vi "SerialEngine.vi"() -> ()   [LabVIEW 2011]
uses:
  Tushars Events/Software/Modules/EventClient_ObjectReference.ctl
  Strict Type Controls/Settings Operation.ctl
  <vilib>/Instr/_visa.llb/VISA Configure Serial Port (Instr).vi
panel:
  out "Quit":bool
  out "error out":errorcluster
  in  "error in (no error)":errorcluster
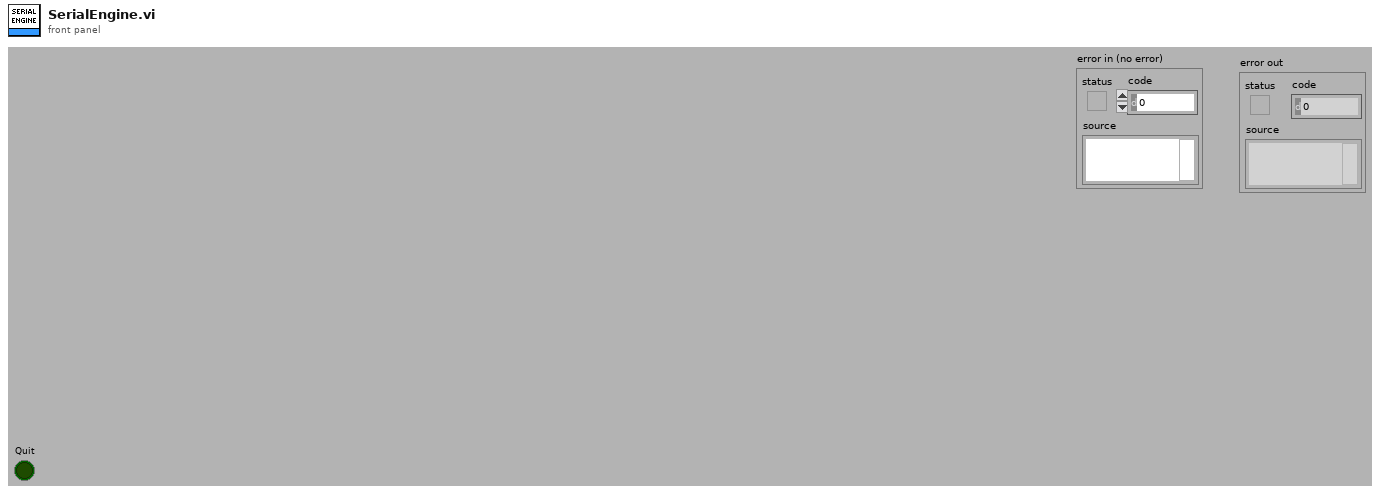
[diagram p1: front panel]
types:
  T1 = typedef "EventClient_ObjectReference.ctl" = refnum<k1>
  T2 = typedef "Settings Operation.ctl" = enum8{"Get Value", "Set Value", "Read File", "Write File", "Write Stored Value"}
  T3 = typedef "Settings.ctl" = cluster{"DMM Settings":cluster{"Port":refnum<visa-resource-name>, "baud rate":u32, "data bits":u16, "stop bits":u16, "parity":enum16{"None", "Odd", "Even", "Mark", "Space"}, "flow control":enum16{"None", "XON/XOFF", "RTS/CTS", "XON/XOFF & RTS/CTS", "DTR/DSR", "XON/XOFF & DTR/DSR"}}, "Modbus Settings":cluster{"Port":refnum<visa-resource-name>, "baud rate":u32, "parity":enum16{"None", "Odd", "Even", "Mark", "Space"}, "flow control":enum16{"None", "XON/XOFF", "RTS/CTS", "XON/XOFF & RTS/CTS", "DTR/DSR", "XON/XOFF & DTR/DSR"}}}
  T4 = enum16{"None", "XON/XOFF", "RTS/CTS", "XON/XOFF & RTS/CTS", "DTR/DSR", "XON/XOFF & DTR/DSR"}
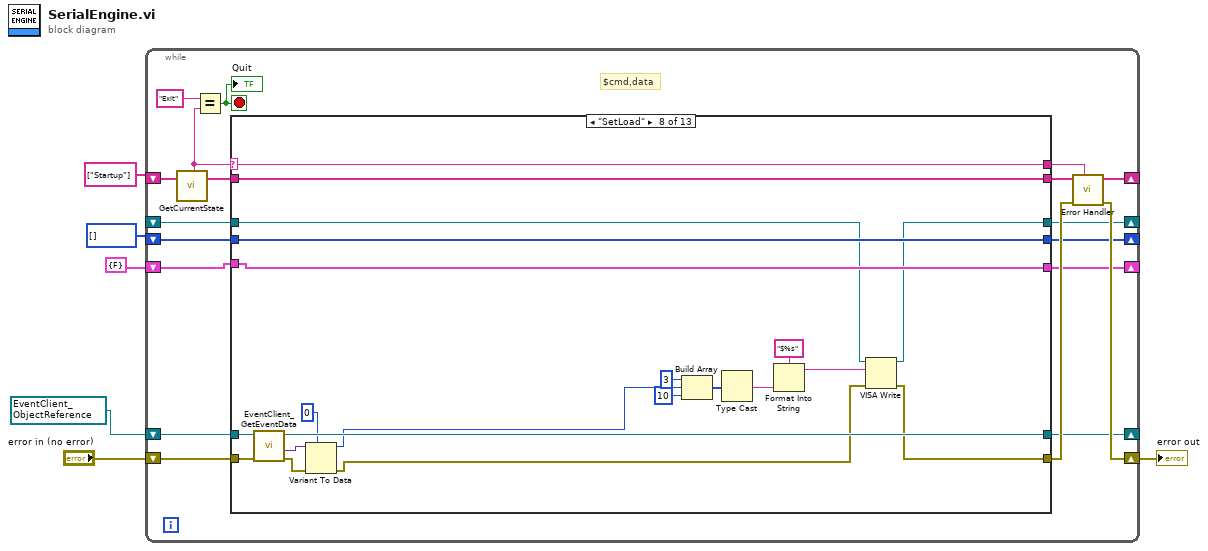
[diagram p0: block diagram]
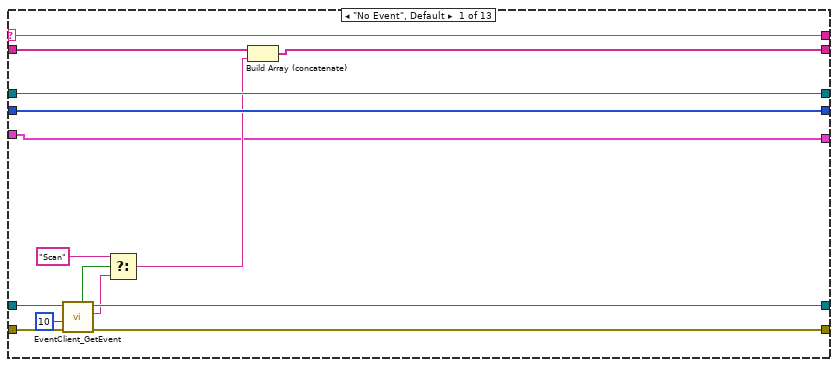
[diagram p2: hidden frame]
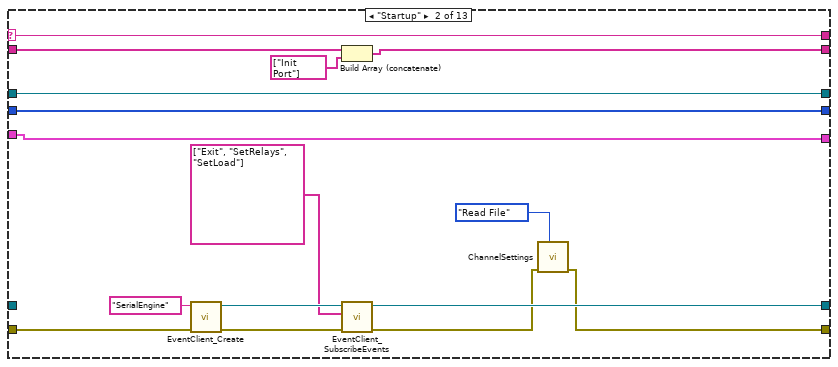
[diagram p3: hidden frame]
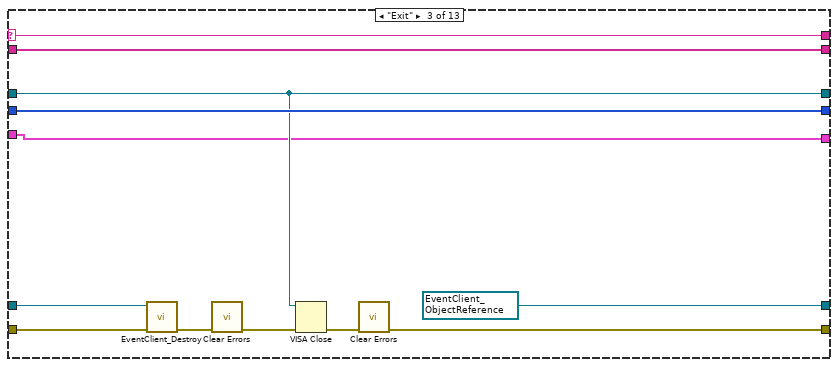
[diagram p4: hidden frame]
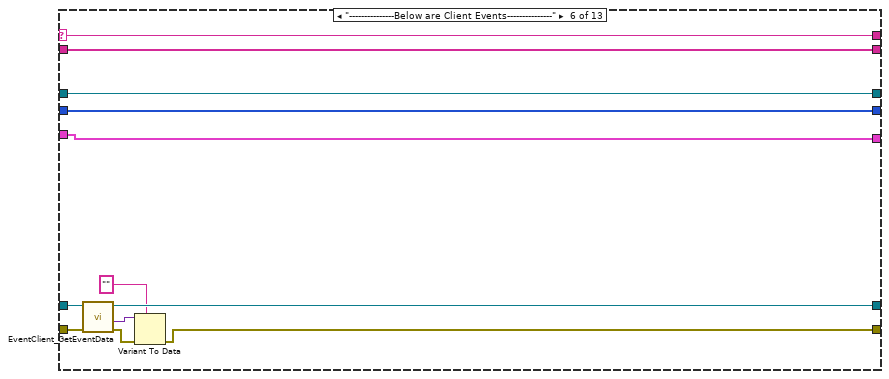
[diagram p7: hidden frame]
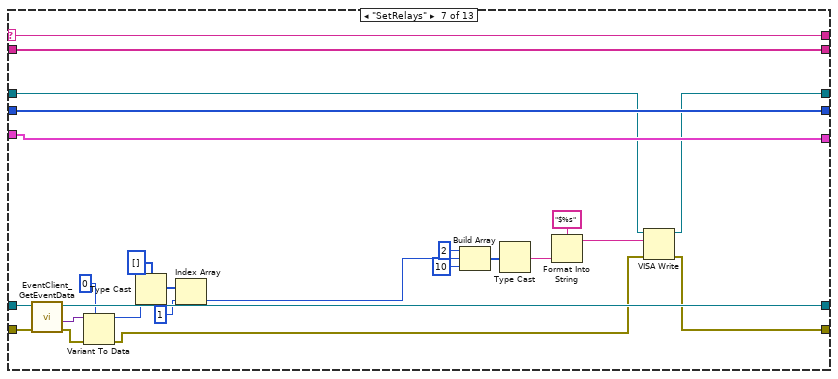
[diagram p8: hidden frame]
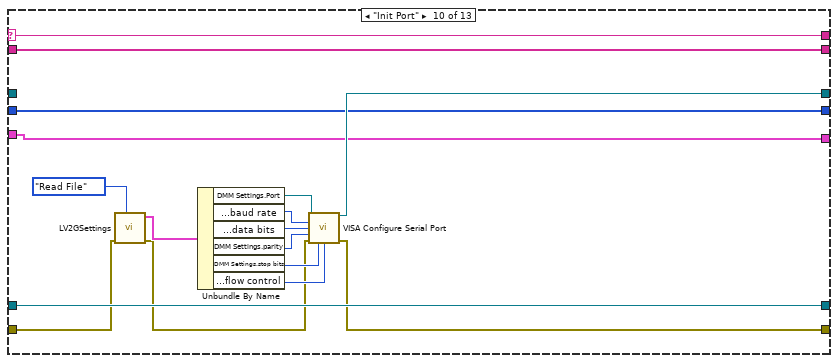
[diagram p10: hidden frame]
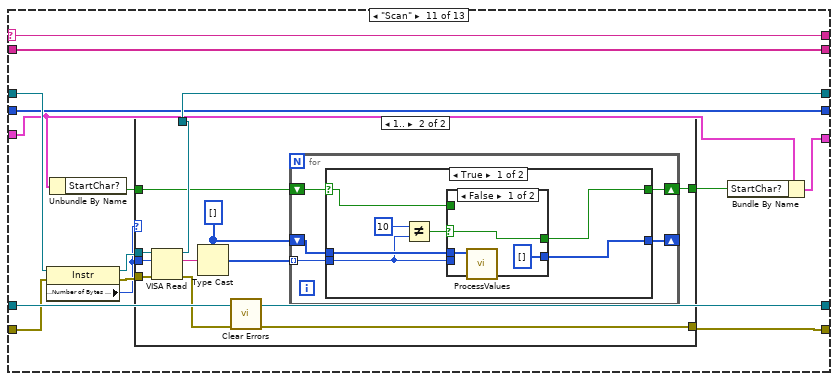
[diagram p11: hidden frame]
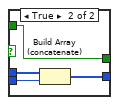
[diagram p13: hidden frame]
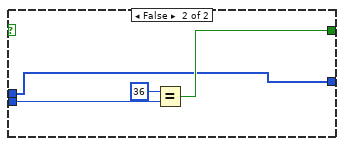
[diagram p14: hidden frame]
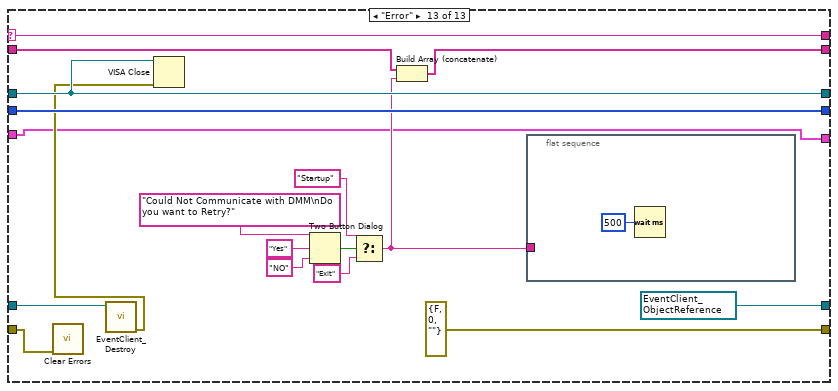
[diagram p16: hidden frame]
diagram:
  w3 = T1 refnum items=["EventClient"] ("reference")
  n1 = while {
    shift-right: [w21] -> _
    shift-left: string[] ["Startup"] ("State Array Out") -> [w25]
    shift-right: [w17] -> w4
    shift-left: "error in (no error)" -> [w18]
    shift-right: [w14] -> _
    shift-left: w3 -> [w13]
    shift-right: [w12] -> _
    shift-left: _ -> [w11]
    shift-right: [w9] -> _
    shift-left: u8[] [] -> [w10]
    shift-right: [w7] -> _
    shift-left: cluster{"StartChar?":bool} {"StartChar?"=FALSE} -> [w8]
    stop <- w22 stop-if-true
    # "$cmd,data"
    n2 = call "GetCurrentState.vi"("State Array In"=w25) -> ("Current State"=w15:string, "State Array Out"=w24:string[])  [unwired: 1 in, 16 out]
    n3 = Equal?(x="Exit", y=w15) -> (x = y?=w22:bool)
    "Quit" <- w22
    n4 = case shown="\"SetLoad\"" w15 {
      selector: w15 -> [w40 w56 w68 w74 w81 w93 w118 w139 w146 w163 w178 w223 w241]
      tunnel: w24 -> [w33 w55 w67 w75 w82 w94 w119 w140 w147 w164 w179 w222 w237]
      tunnel: [w35 w54 w67 w75 w82 w94 w119 w140 w147 w164 w179 w222 w236] -> w20
      tunnel: [w37 w43 w58 w73 w80 w89 w108 w129 w145 w152 w171 w221 errorcluster {"status"=FALSE, "code"=0, "source"=""} ("error in (no error)")] -> w16
      tunnel: [w40 w56 w68 w74 w81 w93 w118 w139 w146 w163 w178 w223 w241] -> w19
      tunnel: w18 -> [w38 w52 w65 w73 w80 w91 w116 w137 w145 w161 w172 w221 w226]
      tunnel: [w36 w49 w64 w72 w79 w87 w113 w134 w144 w162 w177 w220 w227] -> w14
      tunnel: w13 -> [w39 _ w66 w72 w79 w92 w117 w138 w144 w162 w177 w220 w228]
      tunnel: [w32 w46 w62 w71 w78 w86 w106 w127 w143 w151 w173 w219 w238] -> w12
      tunnel: w11 -> [w32 w46 w62 w71 w78 w86 w107 w128 w143 _ w174 w219 w238]
      tunnel: w10 -> [w31 w45 w63 w70 w77 w85 w112 w133 w142 w150 w170 w218 w239]
      tunnel: [w31 w45 w63 w70 w77 w85 w112 w133 w142 w150 w170 w218 w239] -> w9
      tunnel: w8 -> [w26 w41 w57 w69 w76 w83 w111 w132 w141 w149 w167 w217 w224]
      tunnel: [w26 w41 w57 w69 w76 w83 w111 w132 w141 w149 w166 w217 w224] -> w7
      frame "No Event", Default {
        n5 = call "EventClient_GetEvent.vi"("error in (no error)"=w38, "timeout in ms (-1)"=10, "reference"=w39) -> ("error out"=w37:errorcluster, "Name"=w28:string, "reference out"=w36:T1, "timed out?"=w30:bool)  [unwired: 5 out]
        n6 = Select(t="Scan" ("x"), s=w30, f=w28) -> (s? t:f=w27:string)
        n7 = Build Array (concatenate)(w33, w27) -> (w35:string[])
      }
      frame "Startup" {
        n8 = call "EventClient_Create.vi"("error in (no error)"=w52, "Instance Name"="SerialEngine") -> ("error out"=w51:errorcluster, "reference"=w50:T1)  [unwired: 8 out]
        n9 = Build Array (concatenate)(w55, string[] ["Init Port"] ("State Array Out")) -> (w54:string[])
        n10 = call "EventClient_SubscribeEvents.vi"("error in (no error)"=w51, "Events"=string[] ["Exit", "SetRelays", "SetLoad"], "reference"=w50) -> ("error out"=w44:errorcluster, "reference out"=w49:T1)  [unwired: 7 out]
        n11 = call "ChannelSettings.vi"("Operation"=Settings_Operation."Read File", "error in (no error)"=w44) -> ("error out"=w43:errorcluster)  [unwired: 4 in, 4 out]
      }
      frame "Exit" {
        w64 = T1 refnum items=["EventClient"] ("reference out")
        n12 = call "EventClient_Destroy.vi"("error in (no error)"=w65, "reference"=w66) -> ("error out"=w61:errorcluster)  [unwired: 9 out]
        n13 = call <vilib>:"Clear Errors.vi"("error in (no error)"=w61) -> ("error out"=w60:errorcluster)  [unwired: 6 out]
        n14 = VISA Close(VISA resource name=w62, error in (no error)=w60) -> (error out=w59:errorcluster)
        n15 = call <vilib>:"Clear Errors.vi"("error in (no error)"=w59) -> ("error out"=w58:errorcluster)  [unwired: 6 out]
      }
      frame "---------------Below are UI Events---------------" {
        # "This State will never Execute\nIt is added just for improving code readability please do not remove this case"
      }
      frame "---------------Below are Menu Events---------------" {
        # "This State will never Execute\nIt is added just for improving code readability please do not remove this case"
      }
      frame "---------------Below are Client Events---------------" {
        n16 = call "EventClient_GetEventData.vi"("error in (no error)"=w91, "reference"=w92) -> ("error out"=w90:errorcluster, "Data"=w88:variant, "reference out"=w87:T1)  [unwired: 7 out]
        n17 = Variant To Data(error in=w90, type="", Variant=w88) -> (error out=w89:errorcluster)  [unwired: 1 out]
      }
      frame "SetRelays" {
        n18 = call "EventClient_GetEventData.vi"("error in (no error)"=w116, "reference"=w117) -> ("error out"=w115:errorcluster, "Data"=w114:variant, "reference out"=w113:T1)  [unwired: 7 out]
        n19 = Variant To Data(error in=w115, type=u16 0, Variant=w114) -> (data=w100:u16, error out=w109:errorcluster)
        n20 = Type Cast(type=u8[] [], x=w100) -> (*(type *) &x=w99:u8[])
        n21 = Index Array(array=w99, index=1) -> (element=w96:u8)
        n22 = Build Array(u8 2 ("element"), w96, u8 10 ("element")) -> (w103:u8[])
        n23 = Type Cast(x=w103) -> (*(type *) &x=w104:string)  [unwired: 1 in]
        n24 = Format Into String(format string="$%s", w104) -> (resulting string=w102:string)  [unwired: 2 in, 1 out]
        n25 = VISA Write(VISA resource name=w107, write buffer=w102, error in (no error)=w109) -> (VISA resource name out=w106:refnum<visa-resource-name>, error out=w108:errorcluster)  [unwired: 1 out]
      }
      frame "SetLoad" {
        n26 = call "EventClient_GetEventData.vi"("error in (no error)"=w137, "reference"=w138) -> ("error out"=w136:errorcluster, "Data"=w135:variant, "reference out"=w134:T1)  [unwired: 7 out]
        n27 = Variant To Data(error in=w136, type=u8 0, Variant=w135) -> (data=w120:u8, error out=w130:errorcluster)
        n28 = Build Array(u8 3 ("element"), w120, u8 10 ("element")) -> (w124:u8[])
        n29 = Type Cast(x=w124) -> (*(type *) &x=w125:string)  [unwired: 1 in]
        n30 = Format Into String(format string="$%s", w125) -> (resulting string=w123:string)  [unwired: 2 in, 1 out]
        n31 = VISA Write(VISA resource name=w128, write buffer=w123, error in (no error)=w130) -> (VISA resource name out=w127:refnum<visa-resource-name>, error out=w129:errorcluster)  [unwired: 1 out]
      }
      frame "---------------Below are Subroutine states---------------" {
      }
      frame "Init Port" {
        n32 = call "LV2GSettings.vi"("Operation"=Settings_Operation."Read File", "error in (no error)"=w161) -> ("error out"=w153:errorcluster, "Settings out"=w159:T3)  [unwired: 1 in, 7 out]
        n33 = Unbundle By Name(w159) -> ("DMM Settings.Port"=w148:refnum<visa-resource-name>, "DMM Settings.baud rate"=w158:u32, "DMM Settings.data bits"=w157:u16, "DMM Settings.parity"=w156:enum16{"None", "Odd", "Even", "Mark", "Space"}, "DMM Settings.stop bits"=w155:u16, "DMM Settings.flow control"=w154:T4)
        n34 = call-poly "VISA Configure Serial Port"("VISA resource name"=w148, "baud rate (9600)"=w158, "data bits (8)"=w157, "parity (0:none)"=w156, "error in (no error)"=w153, "stop bits (10: 1 bit)"=w155, "flow control (0:none)"=w154) -> ("VISA resource name out"=w151:refnum<visa-resource-name>, "error out"=w152:errorcluster)  [unwired: 7 out]
      }
      frame "Scan" {
        n35 = property class="Instr"(reference=w174, error in=w172) -> (reference out=w175:refnum<visa-resource-name>, error out=w176:errorcluster, "Serial Settings:Number of Bytes at Serial Port"=w169:u32)
        n36 = Unbundle By Name(w167) -> ("StartChar?"=w168:bool)
        n37 = case shown="1.." w169 {
          tunnel: w176 -> [w181 w193]
          tunnel: w169 -> [_ w191]
          tunnel: w175 -> [w182 w190]
          tunnel: [w182 w189] -> w173
          tunnel: [w181 w185] -> w171
          tunnel: w168 -> [w180 w184]
          tunnel: [w180 w183] -> w165
          frame 0, Default {
          }
          frame 1.. {
            w187 = u8[] []
            n38 = VISA Read(VISA resource name=w190, byte count=w191, error in (no error)=w193) -> (VISA resource name out=w189:refnum<visa-resource-name>, read buffer=w192:string, error out=w186:errorcluster)  [unwired: 1 out]
            n39 = Type Cast(type=w187, x=w192) -> (*(type *) &x=w188:u8[])
            n40 = call <vilib>:"Clear Errors.vi"("error in (no error)"=w186) -> ("error out"=w185:errorcluster)  [unwired: 6 in]
            n41 = for {
              tunnel: w188 -> [w198] mode=indexing
              shift-right: [w194] -> _
              shift-left: w187 -> [w197]
              shift-right: [w195] -> w183
              shift-left: w184 -> [w196]
              n42 = case shown="True" w196 {
                selector: w196 -> [w199 _]
                tunnel: w198 -> [w203 w215]
                tunnel: w197 -> [w204 w213]
                tunnel: [w200 w214] -> w195
                tunnel: [w205 w213] -> w194
                frame True {
                  n43 = Not Equal?(x=u8 10, y=w203) -> (x != y?=w201:bool)
                  n44 = case shown="False" w201 {
                    selector: w201 -> [w208 _]
                    tunnel: [u8[] [] w212] -> w205
                    tunnel: w204 -> [w207 w211]
                    tunnel: w203 -> [_ w210]
                    tunnel: [w208 w209] -> w200
                    tunnel: w199 -> [_ w209]
                    frame False {
                      n45 = call "ProcessValues.vi"("ArrayIn"=w207) -> ()  [unwired: 11 in]
                    }
                    frame True {
                      n46 = Build Array (concatenate)(w211, w210) -> (w212:u8[])
                    }
                  }
                }
                frame False {
                  n47 = Equal?(x=u8 36, y=w215) -> (x = y?=w214:bool)
                }
              }
            }
          }
        }
        n48 = Bundle By Name(cluster=w167, "StartChar?"=w165) -> (w166:cluster{"StartChar?":bool})
      }
      frame "---------------Below are Error Handling VIs---------------" {
      }
      frame "Error" {
        w227 = T1 refnum items=["EventClient"] ("reference")
        n49 = call <vilib>:"Clear Errors.vi"("error in (no error)"=w226) -> ()  [unwired: 7 out]
        n50 = call "EventClient_Destroy.vi"("reference"=w228) -> ("error out"=w225:errorcluster)  [unwired: 1 in, 9 out]
        n51 = VISA Close(VISA resource name=w238, error in (no error)=w225) -> ()  [unwired: 1 out]
        n52 = Two Button Dialog(message="Could Not Communicate with DMM\nDo you want to Retry?", 1:"NO" ("F button name (\"Cancel\")"), 2:"Yes" ("T button name (\"OK\")")) -> (T button?=w232:bool)
        n53 = Select(t="Startup" ("String"), s=w232, f="Exit" ("String")) -> (s? t:f=w229:string)
        n54 = Build Array (concatenate)(w237, w229) -> (w236:string[])
        n55 = flat-sequence {
          tunnel: w229 -> [_]
          frame #0 {
            n56 = Wait (ms)(milliseconds to wait=u32 500) -> ()  [unwired: 1 out]
          }
        }
      }
    }
    n57 = call "Error Handler.vi"("Current State"=w19, "error in (no error)"=w16, "Msg Queue In"=w20) -> ("error out"=w17:errorcluster, "Msg Queue Out"=w21:string[])  [unwired: 1 in, 6 out]
  }
  "error out" <- w4
